vi "WPI_Power Get roboRIO Input Voltage and Current.vi"(11 "error in":errorcluster) -> (6 "roboRIO input voltage (V)":dbl, 8 "roboRIO input current (A)":dbl, 15 "error out":errorcluster)   [LabVIEW 2017]
doc: "Returns the voltage and current of the INPUT power on the roboRIO."
uses:
  <vilib>/Utility/error.llb/Error Cluster From Error Code.vi
  <vilib>/rvi/errors/niLvFpgaAdjustHostInterfaceError.vi
  <vilib>/rvi/interface/nirviReadWriteControl/nirviReadWriteControl.xnode
  <vilib>/Rock Robotics/SystemInterfaces/System/FPGA_SystemFRC FPGA Ref.ctl
  NiFpgaLv.dll
  <vilib>/rvi/interface/Simulation/niFpgaSimulationCallBeginRW.vi
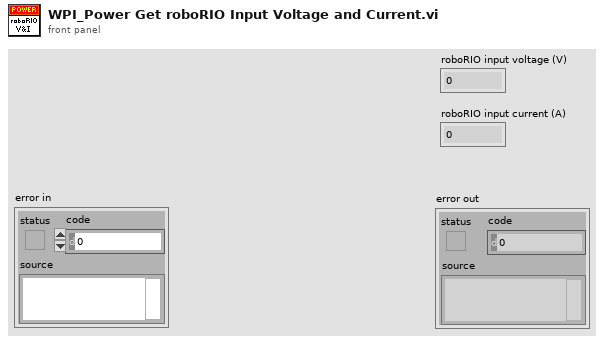
[diagram p1: front panel]
types:
  T1 = typedef "FPGA_SystemFRC FPGA Ref.ctl" = refnum<k20>
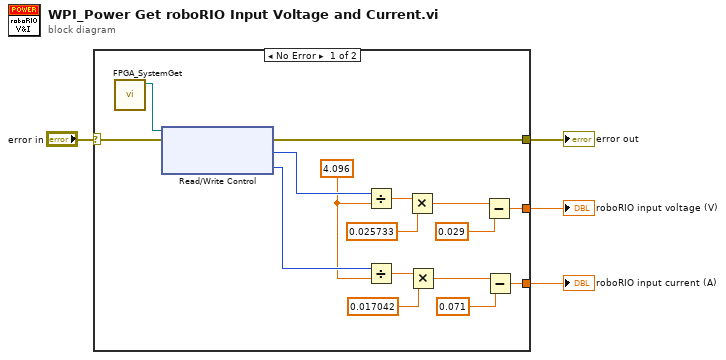
[diagram p0: block diagram]
diagram:
  n1 = case shown="No Error" "error in" {
    selector: "error in" -> [w10 w21]
    tunnel: [w8 w21] -> w3
    tunnel: [w17 _] -> w2
    tunnel: [w13 _] -> w1
    frame No Error {
      w5 = 4.096 ("battery voltage out")
      n2 = call <vilib>:"FPGA_SystemGet.vi"() -> ("FRC FPGA Ref"=w11:T1)  [unwired: 2 in, 9 out]
      n3 = xnode "Read/Write Control"("FPGA VI Reference In"=w11, "error in"=w10) -> ("error out"=w8:errorcluster, "Power.VinVoltage"=w7:u16, "Power.VinCurrent"=w6:u16)  [unwired: 1 out]
      n4 = Divide(x=w7, y=w5) -> (x/y=w12:dbl)
      n5 = Divide(x=w6, y=w5) -> (x/y=w9:dbl)
      n6 = Multiply(x=w12, y=0.025733 ("battery voltage out")) -> (x*y=w19:dbl)
      n7 = Multiply(x=w9, y=0.017042 ("battery voltage out")) -> (x*y=w15:dbl)
      n8 = Subtract(x=w19, y=0.029 ("battery voltage out")) -> (x-y=w17:dbl)
      n9 = Subtract(x=w15, y=0.071 ("battery voltage out")) -> (x-y=w13:dbl)
    }
    frame Error {
    }
  }
  "error out" <- w3
  "roboRIO input voltage (V)" <- w2
  "roboRIO input current (A)" <- w1
